vi "List VIs without Test Coverage.vi"(8 "error in (no error)":errorcluster, 9 "Tests Root":path, 10 "Source Root":path) -> (0 "error out":errorcluster, 1 "Test VIs":path[](array[path]), 2 "VIs without test coverage":string[](array[string]))   [LabVIEW 2009]
uses:
  <userlib>/_OpenG.lib/array/array.llb/Conditional Auto-Indexing Tunnel (String)__ogtk.vi
  <userlib>/_OpenG.lib/file/file.llb/Build Path - File Names Array__ogtk.vi
  <userlib>/_OpenG.lib/file/file.llb/Compare Two Paths - Scalar__ogtk.vi
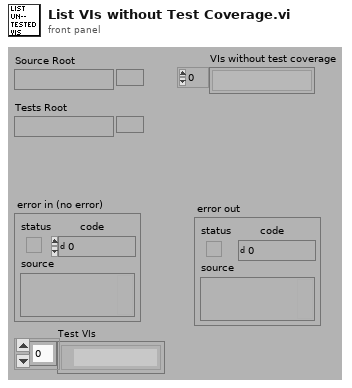
[diagram p1: front panel]
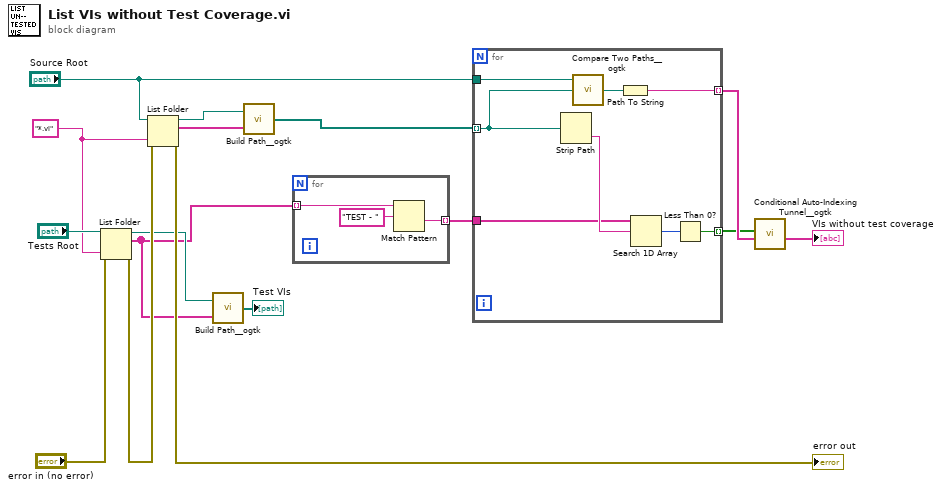
[diagram p0: block diagram]
diagram:
  w9 = "*.vi" ("pattern")
  n1 = List Folder(path="Tests Root", pattern=w9, error in="error in (no error)") -> (path out=w3:path, filenames=w2:string[], error out=w10:errorcluster)  [unwired: 1 in, 1 out]
  n2 = List Folder(path="Source Root", pattern=w9, error in=w10) -> (path out=w7:path, filenames=w5:string[], error out=→"error out":errorcluster)  [unwired: 1 in, 1 out]
  n3 = call-poly <userlib>:"Build Path__ogtk.vi"("name or relative path"=w2, "base path"=w3) -> ("appended path"=→"Test VIs":path[])
  n4 = call-poly <userlib>:"Build Path__ogtk.vi"("name or relative path"=w5, "base path"=w7) -> ("appended path"=w6:path[])
  n5 = for {
    tunnel: w2 -> [w19] mode=indexing
    tunnel: [w17] -> w8 mode=indexing
    n6 = Match Pattern(string=w19, regular expression="TEST - ") -> (after substring=w17:string)  [unwired: 1 in, 3 out]
  }
  n7 = for {
    tunnel: w6 -> [w22] mode=indexing
    tunnel: w8 -> [w26]
    tunnel: [w24] -> w14 mode=indexing
    tunnel: "Source Root" -> [w23]
    tunnel: [w20] -> w15 mode=indexing
    n8 = Strip Path(path=w22) -> (name=w27:string)  [unwired: 1 out]
    n9 = call-poly <userlib>:"Compare Two Paths__ogtk.vi"("path2"=w22, "path1"=w23) -> ("relative path from 1 to 2"=w21:path)  [unwired: 1 in, 2 out]
    n10 = Path To String(path=w21) -> (string=w20:string)
    n11 = Search 1D Array(1D array=w26, element=w27) -> (index of element=w25:i32)  [unwired: 1 in]
    n12 = Less Than 0?(x=w25) -> (x < 0?=w24:bool)
  }
  n13 = call-poly <userlib>:"Conditional Auto-Indexing Tunnel__ogtk.vi"("Array in"=w15, "Elements to keep"=w14) -> ("Filtered Array out"=→"VIs without test coverage":string[])  [unwired: 5 in]
